vi "refgen.vi"(7 "refgen":cluster{"slope":dbl, "period":dbl}, 11 "Qube":refnum<class "Qube.lvclass">) -> (1 "r":dbl, 3 "Qube":refnum<class "Qube.lvclass">)   [LabVIEW 2020, in "Qube.lvclass"]
uses:
  Qube.lvclass
  Qube.lvclass/Qube.ctl
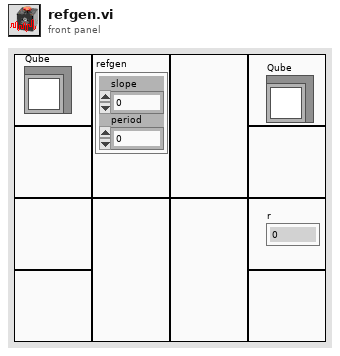
[diagram p1: front panel]
types:
  T1 = typedef "Qube.lvclass/mode.ctl" = enum16{"Control", "Identify"}
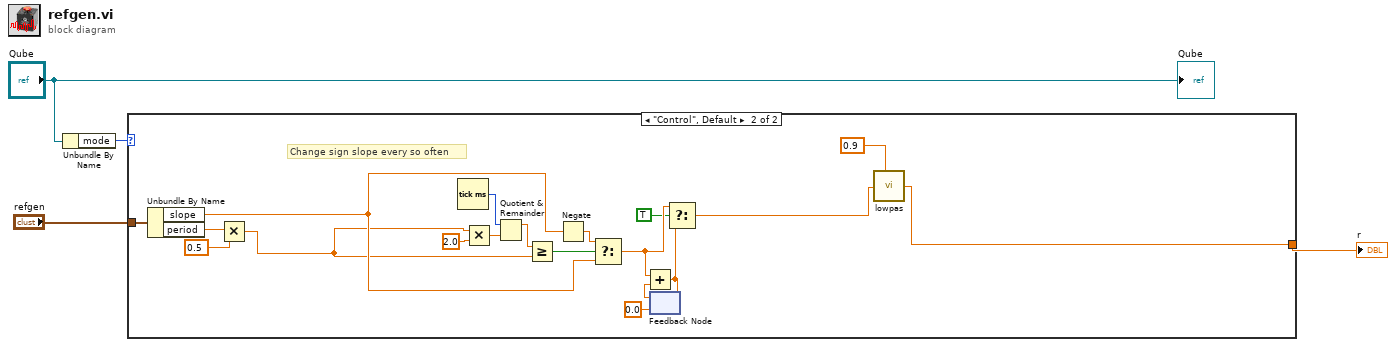
[diagram p0: block diagram]
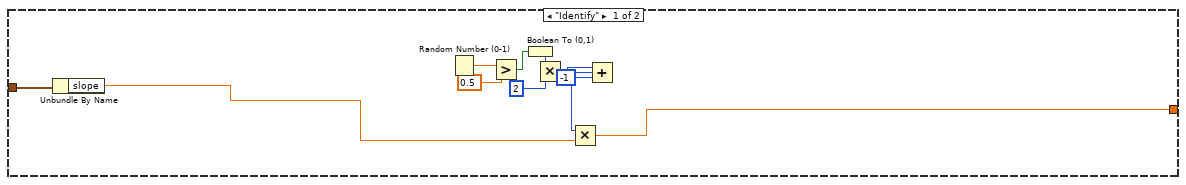
[diagram p2: hidden frame]
diagram:
  n1 = Unbundle By Name("Qube") -> ("mode"=w3:T1)
  n2 = case shown="\"Control\", Default" w3 {
    tunnel: [w7 w17] -> w4
    tunnel: "refgen" -> [w15 w34]
    frame "Identify" {
      n3 = Unbundle By Name(w15) -> ("slope"=w8:dbl)
      n4 = Random Number (0-1)() -> (number: 0 to 1=w6:dbl)
      n5 = Greater?(x=w6, y=0.5) -> (0:w13:bool)
      n6 = Boolean To (0,1)(Boolean=w13) -> (0, 1=w12:i16)
      n7 = Multiply(x=w12, y=i16 2) -> (x*y=w11:i16)
      n8 = Add(x=w11, y=i16 -1) -> (x+y=w5:i16)
      n9 = Multiply(x=w5, y=w8) -> (x*y=w7:dbl)
    }
    frame "Control", Default {
      # "Change sign slope every so often"
      n10 = Unbundle By Name(w34) -> ("slope"=w27:dbl, "period"=w26:dbl)
      n11 = Multiply(x=w26, y=0.5) -> (x*y=w22:dbl)
      n12 = Tick Count (ms)() -> (millisecond timer value=w33:u32)
      n13 = Multiply(x=w22, y=2.0) -> (x*y=w32:dbl)
      n14 = Quotient & Remainder(x=w33, y=w32) -> (x-y*floor(x/y)=w30:dbl)  [unwired: 1 out]
      n15 = Greater Or Equal?(x=w30, y=w22) -> (x >= y?=w29:bool)
      n16 = Negate(x=w27) -> (-x=w28:dbl)
      n17 = Select(t=w28, s=w29, f=w27) -> (s? t:f=w20:dbl)
      n18 = feedback #1(0.0) -> (w24:dbl)
      n19 = Add(x=w20, y=w24) -> (x+y=w21:dbl)
      n20 = feedback-in #1(w21) -> ()
      n21 = Select(t=w20, s=TRUE, f=w21) -> (s? t:f=w18:dbl)
      n22 = call "lowpas.vi"("alpha"=0.9, "x"=w18) -> ("Numeric"=w17:dbl)  [unwired: 5 in]
    }
  }
  "r" <- w4
  "Qube" <- "Qube"
